vi "Ejecutor_Test.vi"() -> ()   [LabVIEW 2019]
panel:
  in  "Tab Control":enum32{"Page 1", "Page 2"}(tab)
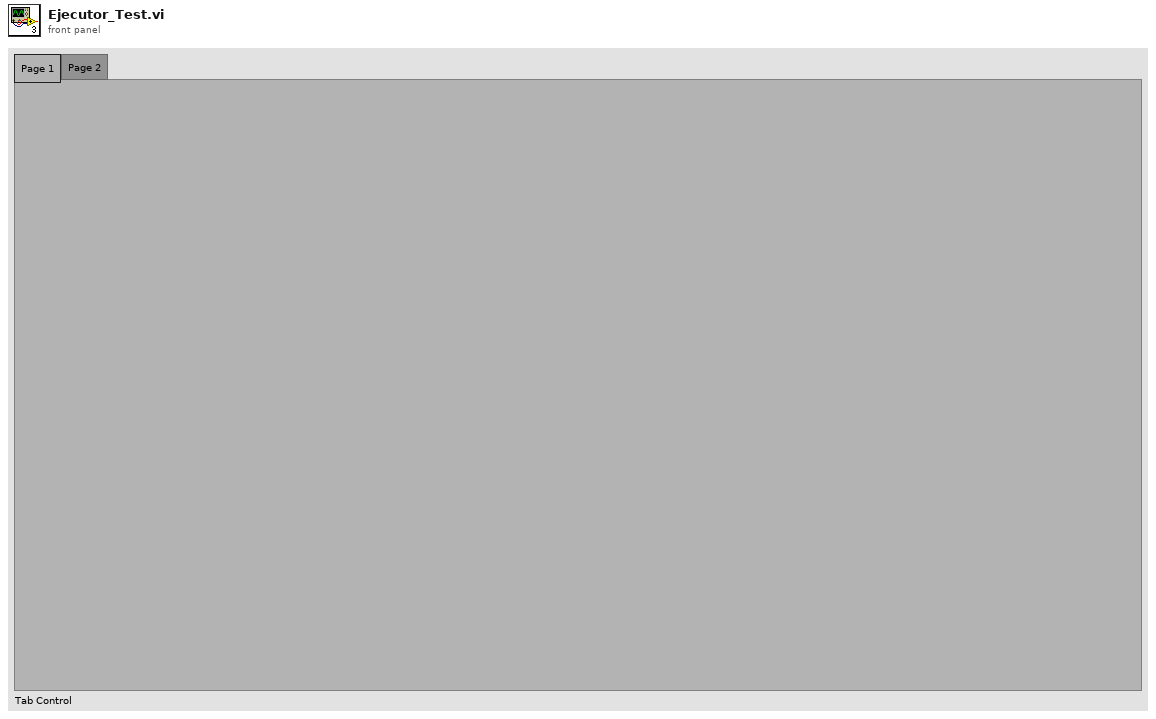
[diagram p1: front panel]
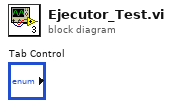
[diagram p0: block diagram]
diagram:
